vi "lab10_target_2_subvi1.vi"(8 "error in (no error)":errorcluster, 10 "event_id":dbl, 11 "start_time":dbl) -> (0 "error out":errorcluster, 3 "Boolean":bool)   [LabVIEW 2020]
uses:
  <vilib>/measure/NI_MABase.lvlib
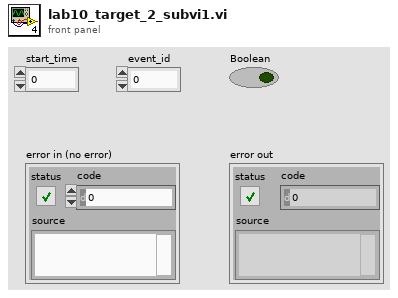
[diagram p1: front panel]
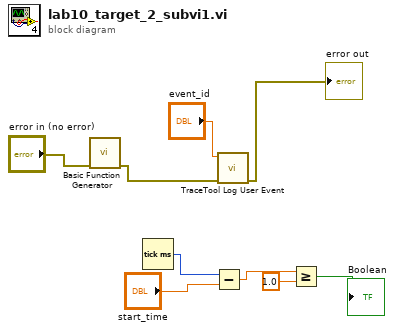
[diagram p0: block diagram]
diagram:
  n1 = call <vilib>:"Basic Function Generator.vi"("error in (no error)"="error in (no error)") -> ("error out"=w8:errorcluster)  [unwired: 8 in, 2 out]
  n2 = Tick Count (ms)() -> (millisecond timer value=w2:u32)
  n3 = Subtract(x=w2, y="start_time") -> (x-y=w4:dbl)
  n4 = call <vilib>:"TraceTool Log User Event.vi"("error in (no error)"=w8, "Event ID (0-255)"="event_id") -> ("error out"=→"error out":errorcluster)  [unwired: 9 in]
  n5 = Greater Or Equal?(x=w4, y=1.0) -> (x >= y?=→"Boolean":bool)
